vi "MouseclickLB.vi"(9 "nMilliseconds":i32=2000, 10 "error in (no error)":errorcluster, 11 "Click":T1(ring)) -> (2 "error out":errorcluster)   [LabVIEW 2014]
panel:
  in  "AutoItX3Lib.IAutoItX3":refnum<k7>
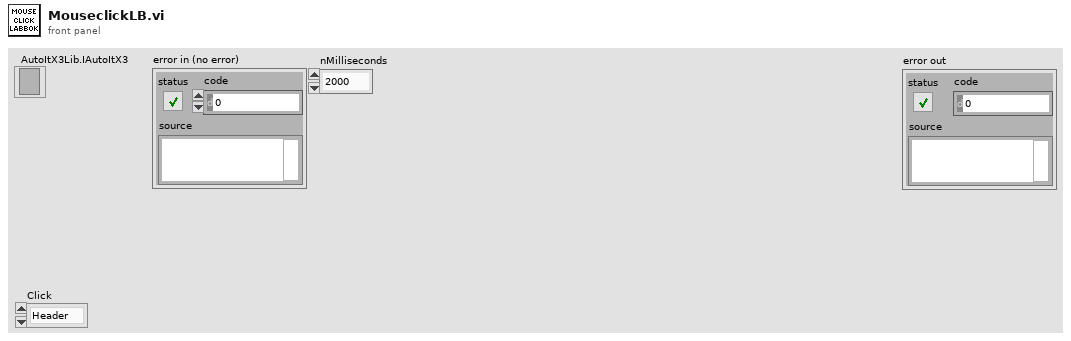
[diagram p1: front panel]
types:
  T1 = enum16{"Header", "TOPO", "STS", "GRID", "GRIDCloud"}
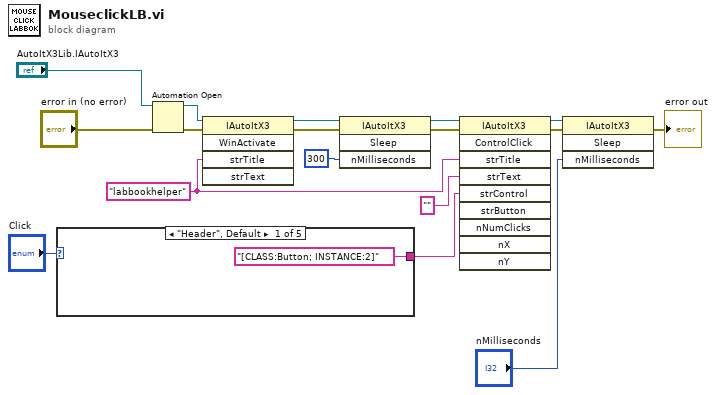
[diagram p0: block diagram]
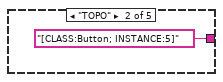
[diagram p2: hidden frame]
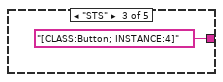
[diagram p3: hidden frame]
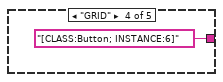
[diagram p4: hidden frame]
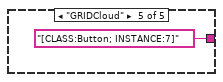
[diagram p5: hidden frame]
diagram:
  w6 = "labbookhelper" ("strTitle")
  n1 = case shown="\"Header\", Default" "Click" {
    tunnel: ["[CLASS:Button; INSTANCE:2]" ("strControl") "[CLASS:Button; INSTANCE:5]" ("strControl") "[CLASS:Button; INSTANCE:4]" ("strControl") "[CLASS:Button; INSTANCE:6]" ("strControl") "[CLASS:Button; INSTANCE:7]" ("strControl")] -> w9
    frame "Header", Default {
    }
    frame "TOPO" {
    }
    frame "STS" {
    }
    frame "GRID" {
    }
    frame "GRIDCloud" {
    }
  }
  n2 = Automation Open(error in (no error)="error in (no error)", Automation Refnum="AutoItX3Lib.IAutoItX3") -> (Automation Refnum=w8:refnum<k7>, error out=w7:errorcluster)  [unwired: 2 in]
  n3 = invoke class="IAutoItX3" method="WinActivate"(reference=w8, error in=w7, "strTitle"=w6) -> (reference out=w5:refnum<k7>, error out=w2:errorcluster)  [unwired: 2 in, 3 out]
  n4 = invoke class="IAutoItX3" method="Sleep"(reference=w5, error in=w2, "nMilliseconds"=300) -> (reference out=w4:refnum<k7>, error out=w3:errorcluster)  [unwired: 1 in, 2 out]
  n5 = invoke class="IAutoItX3" method="ControlClick"(reference=w4, error in=w3, "strTitle"=w6, "strText"="", "strControl"=w9) -> (reference out=w15:refnum<k7>, error out=w14:errorcluster)  [unwired: 5 in, 8 out]
  n6 = invoke class="IAutoItX3" method="Sleep"(reference=w15, error in=w14, "nMilliseconds"="nMilliseconds") -> (error out=→"error out":errorcluster)  [unwired: 1 in, 3 out]
